vi "Configure Modules from Hardware.vi"() -> ()   [LabVIEW 2020]
uses:
  NationalInstruments.VeriStand.SystemDefinitionAPI
  <vilib>/addons/VeriStand Custom Device Scripting APIs/SLSC Switch/VeriStand SLSC Scripting API/VeriStand SLSC Scripting.lvlib
  <vilib>/addons/VeriStand Custom Device Scripting APIs/SLSC Switch/Scripting/SLSC Switch Scripting.lvlib
  SLSC Switch Examples.lvlib
panel:
  in  "SLSC Chassis Name or IP":string="slsc-12001-00000000"
  in  "Controller Name":string="Controller"
  in  "SLSC Modules":refnum<k21>[](array[refnum])
  in  "Output System Definition file":path=path "System Definition Files/Scripted SLSC Switch.nivssdf"
  in  "Input System Definition File":path=path "System Definition Files/Base with SLSC Chassis.nivssdf"
  # "Overview: Demonstrates using the SLSC Switch custom device scripting API to configure instances of the custom device to reflect real hardware.\n\nInstructions:\n1. Browse to the system definition file to be used as input.\n2. Browse to a path to save the system definition file as output. This may be the same as the input file.\n3. Set the name of the controller in the system definition file that contains the SLSC Chassis\nand the SLSC Chassis identifier used in the system definition file. \n4. Select the SLSC modules to script into the system definition file.\n5. Run the VI and verify its results."
  # "System Definition Files"
  # "SLSC Chassis"
  # "SLSC Switch Modules"
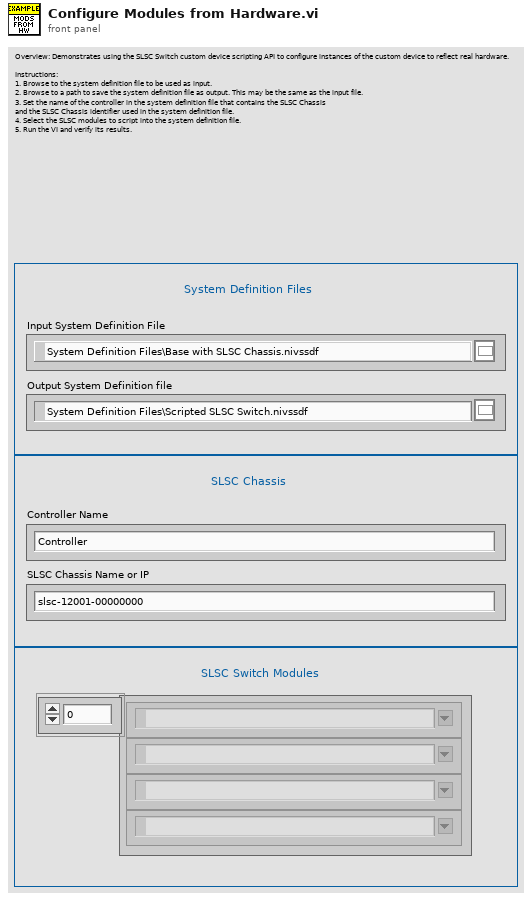
[diagram p1: front panel]
types:
  T1 = typedef "Custom Device API.lvlib/Custom Device Item Ref.ctl" = u64
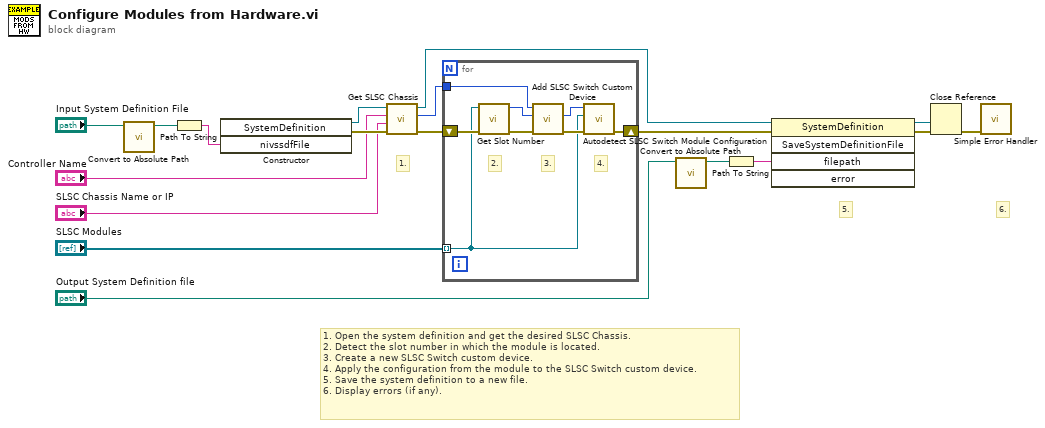
[diagram p0: block diagram]
diagram:
  # "6."
  # "5."
  # "1."
  # "1. Open the system definition and get the desired SLSC Chassis.\n2. Detect the slot number in which the module is located.\n3. Create a new SLSC Switch custom device.\n4. Apply the configuration from the module to the SLSC Switch custom device.\n5. Save the system definition to a new file.\n6. Display errors (if any)."
  n1 = call "Convert to Absolute Path.vi"("System Definition File"="Input System Definition File") -> ("Absolute Path"=w2:path)  [unwired: 10 in]
  n2 = Path To String(path=w2) -> (string=w11:string)
  n3 = constructor class="SystemDefinition"("nivssdfFile"=w11) -> (reference out=w9:refnum<k24>, error out=w10:errorcluster)  [unwired: 3 in, 2 out]
  n4 = call <vilib>:"Get SLSC Chassis.vi"("error in (no error)"=w10, "SLSC Chassis Name or IP"="SLSC Chassis Name or IP", "Target Name"="Controller Name", "SysDef in"=w9) -> ("error out"=w8:errorcluster, "SLSC Chassis"=w7:u64, "SysDef out"=w6:refnum<k24>)  [unwired: 4 in, 1 out]
  n5 = for {
    tunnel: "SLSC Modules" -> [w19] mode=indexing
    shift-right: [w24] -> w14
    shift-left: w8 -> [w22]
    tunnel: w7 -> [w26]
    # "4."
    # "3."
    # "2."
    n6 = call "Get Slot Number.vi"("error in (no error)"=w22, "SLSC Device"=w19) -> ("error out"=w21:errorcluster, "slot number"=w20:u32)  [unwired: 7 in]
    n7 = call <vilib>:"Add SLSC Switch Custom Device.vi"("error in"=w21, "slot number"=w20, "slsc chassis in"=w26) -> ("error out"=w25:errorcluster, "slsc switch custom device"=w23:T1)  [unwired: 6 in, 1 out]
    n8 = call <vilib>:"Autodetect SLSC Switch Module Configuration.vi"("error in"=w25, "slsc module"=w19, "slsc switch custom device in"=w23) -> ("error out"=w24:errorcluster)  [unwired: 7 in, 1 out]
  }
  n9 = call "Convert to Absolute Path.vi"("System Definition File"="Output System Definition file") -> ("Absolute Path"=w1:path)  [unwired: 10 in]
  n10 = Path To String(path=w1) -> (string=w18:string)
  n11 = invoke class="SystemDefinition" method="SaveSystemDefinitionFile"(reference=w6, error in=w14, "filepath"=w18) -> (reference out=w16:refnum<k24>, error out=w17:errorcluster)  [unwired: 2 in, 3 out]
  n12 = Close Reference(reference=w16, error in (no error)=w17) -> (error out=w12:errorcluster)
  n13 = call <vilib>:"Simple Error Handler.vi"("error in (no error)"=w12) -> ()  [unwired: 1 in, 8 out]
